vi "FeuRouge.vi"() -> ()   [LabVIEW 2018]
uses:
  FeuControle.vi
panel:
  in  "stop":bool
  out "Vert":bool
  out "Orange":bool
  out "Rouge":bool
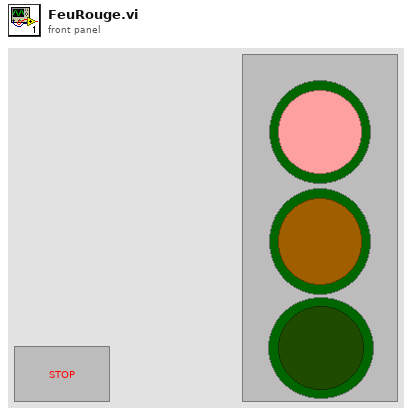
[diagram p1: front panel]
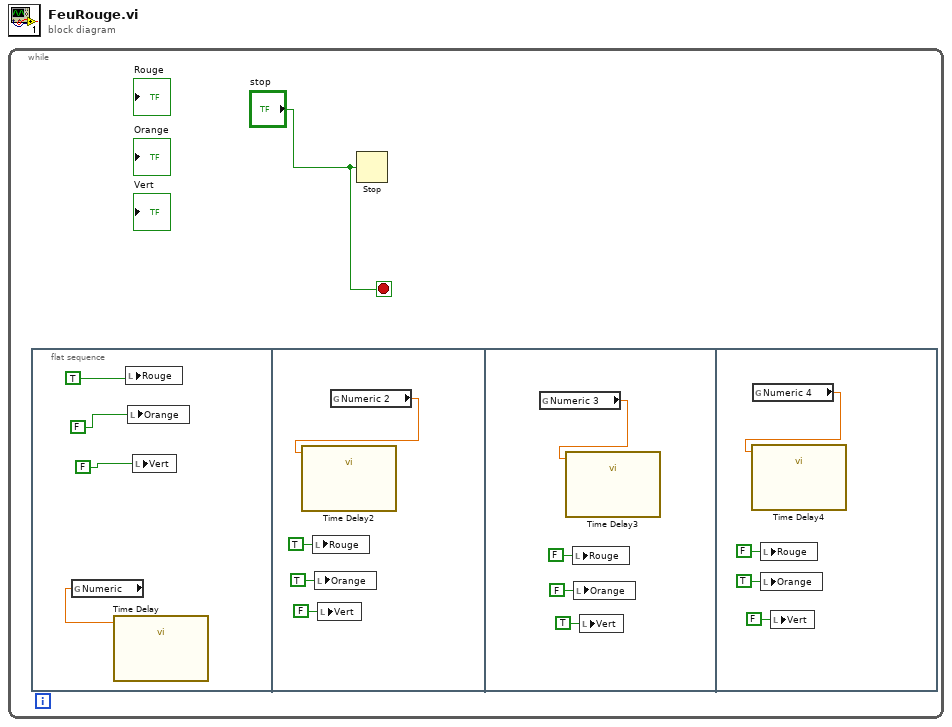
[diagram p0: block diagram]
diagram:
  n1 = while {
    stop <- "stop" stop-if-true
    n2 = flat-sequence {
      frame #0 {
        n3 = global read "FeuControle.vi" "Numeric"() -> (w5:dbl)
        n4 = call "Time Delay"("Delay Time (s)"=w5) -> ()  [unwired: 10 in, 1 out]
        n5 = local write "Rouge"(TRUE) -> ()
        n6 = local write "Orange"(FALSE) -> ()
        n7 = local write "Vert"(FALSE) -> ()
      }
      frame #1 {
        n8 = local write "Rouge"(TRUE ("Rouge")) -> ()
        n9 = local write "Orange"(TRUE ("Orange")) -> ()
        n10 = local write "Vert"(FALSE ("Vert")) -> ()
        n11 = global read "FeuControle.vi" "Numeric 2"() -> (w9:dbl)
        n12 = call "Time Delay2"("Delay Time (s)"=w9) -> ()  [unwired: 10 in, 1 out]
      }
      frame #2 {
        n13 = global read "FeuControle.vi" "Numeric 3"() -> (w13:dbl)
        n14 = call "Time Delay3"("Delay Time (s)"=w13) -> ()  [unwired: 10 in, 1 out]
        n15 = local write "Rouge"(FALSE ("Rouge")) -> ()
        n16 = local write "Orange"(FALSE ("Orange")) -> ()
        n17 = local write "Vert"(TRUE ("Vert")) -> ()
      }
      frame #3 {
        n18 = global read "FeuControle.vi" "Numeric 4"() -> (w17:dbl)
        n19 = call "Time Delay4"("Delay Time (s)"=w17) -> ()  [unwired: 10 in, 1 out]
        n20 = local write "Rouge"(FALSE ("Rouge")) -> ()
        n21 = local write "Orange"(TRUE ("Orange")) -> ()
        n22 = local write "Vert"(FALSE ("Vert")) -> ()
      }
    }
    n23 = Stop(stop? (T)="stop") -> ()
  }
